vi "samplesAvailable.vi"(8 "error in (no error)":errorcluster, 11 "RTDisplacement in":refnum<class "RTDisplacement.lvclass">) -> (0 "error out":errorcluster, 2 "SamplesAvailable":bool, 3 "RTDisplacement out":refnum<class "RTDisplacement.lvclass">)   [LabVIEW 2016]
uses:
  Common_RT_FPGA/IReadU64FIFO/IReadU64FIFO.lvclass
  RTDisplacement.lvclass
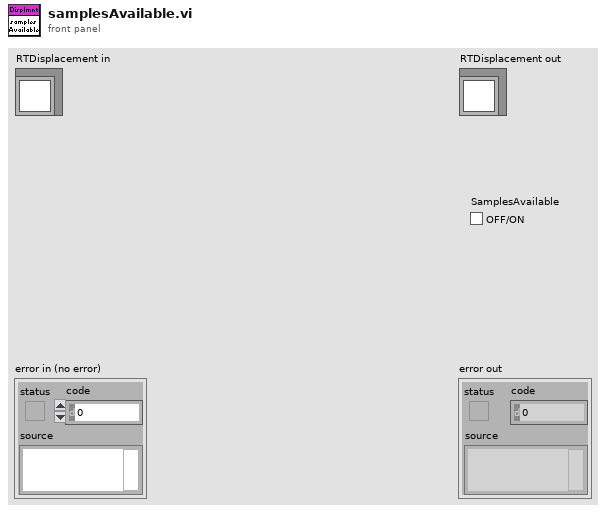
[diagram p1: front panel]
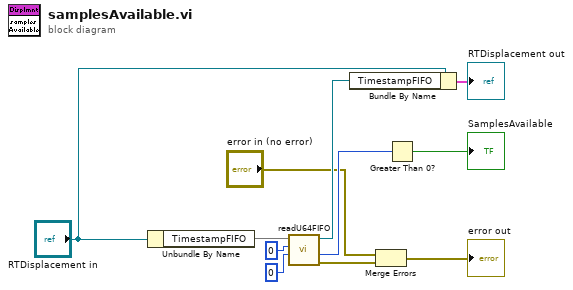
[diagram p0: block diagram]
diagram:
  n1 = Unbundle By Name("RTDisplacement in") -> ("TimestampFIFO"=w9)
  n2 = call-dynamic "readU64FIFO.vi"("Timeout"=0, "NumberOfElements"=u32 0, "IReadU64FIFO in"=w9) -> ("error out"=w3:errorcluster, "ElementsRemaining"=w6:u32, "IReadU64FIFO out"=w4:refnum<class "IReadU64FIFO.lvclass">)  [unwired: 5 in, 1 out]
  n3 = Bundle By Name(cluster="RTDisplacement in", "TimestampFIFO"=w4) -> (→"RTDisplacement out":cluster{})
  n4 = Merge Errors("error in (no error)", w3) -> (→"error out":errorcluster)
  n5 = Greater Than 0?(x=w6) -> (x > 0?=→"SamplesAvailable":bool)
